vi "Create Database.vi"(8 "error in (no error)":errorcluster, 10 "Database Configuration":T1={"Interface"="CAN1", "CAN Cluster"={"Baud Rate"=125000, "Comment"="", "Name"="CAN_Cluster"}, "CAN Frame"={"Frame name"="frame1", "Identifier"=1, "Payload Length"=8, "Timing Type"=1, "Transmit Time"=0.0, "Extended Identifier?"=FALSE, "Comment"=""}, "Signal Cluster"={"Signal name"="signal", "Scaling Factor"=1.0, "Scaling Offset"=0.0, "Maximum Value"=256.0, "Minimum Value"=0.0, "Default Value"=0.0, "Unit"="V", "Start Bit"=0, "Number of Bits"=8, "Data Type"=1, "Byte Order"=0, "Comment"=""}, "Session Type (All Single Point)"=enum."Signal Input"} {"Signal Cluster"."Byte Order" items=["Little Endian", "Big Endian"]; "Signal Cluster"."Data Type" items=["Signed", "Unsigned", "IEEE Float"]; "CAN Frame"."Timing Type" items=["Cyclic Data", "Event Data", "Cyclic Remote", "Event Remote"]}, 11 "PXI 8513 in":refnum<class "PXI 8513.lvclass">) -> (0 "error out":errorcluster, 3 "PXI 8513 out":refnum<class "PXI 8513.lvclass">)   [LabVIEW 2016, in "CAN.lvlib" / "PXI 8513.lvclass"]
uses:
  PXI 8513.lvclass
  CAN Database Configuration.ctl
  C:/Program Files (x86)/National Instruments/LabVIEW 2016/examples/nixnet/examples.llb/NI-XNET Example Control - CAN Cluster.ctl
  C:/Program Files (x86)/National Instruments/LabVIEW 2016/examples/nixnet/examples.llb/NI-XNET Example Control - CAN Frame.ctl
  C:/Program Files (x86)/National Instruments/LabVIEW 2016/examples/nixnet/examples.llb/NI-XNET Example Control - Signal.ctl
  PXI 8513.lvclass/PXI 8513.ctl
  <vilib>/xnet/xnet.llb/XNET Create Session (Signal Input Single-point).vi
  <vilib>/xnet/xnet.llb/XNET Create Session (Signal Output Single-point).vi
  <vilib>/xnet/xnet.llb/XNET Create Session (Frame Input Single-point).vi
  <vilib>/xnet/xnet.llb/XNET Create Session (Frame Output Single-point).vi
  CAN.lvlib
panel:
  in  "Output Data":dbl=6.0 format="%.2f"
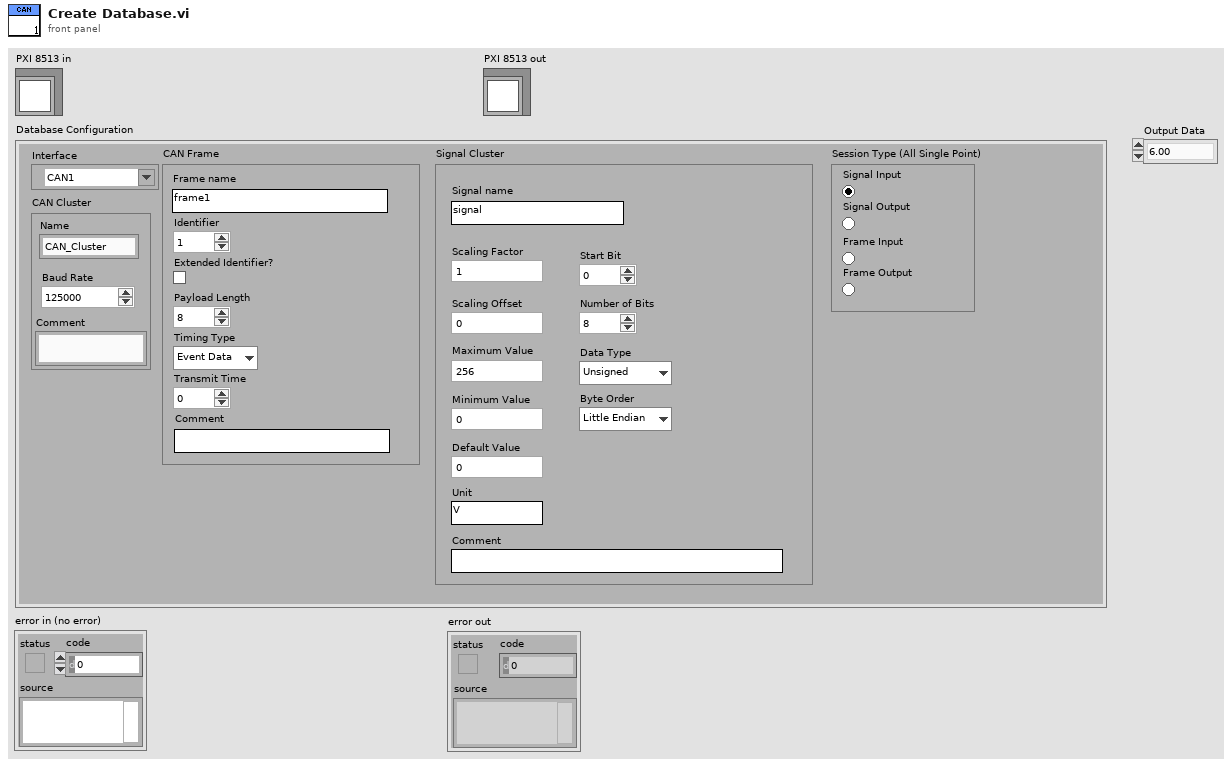
[diagram p1: front panel]
types:
  T1 = typedef "CAN.lvlib/CAN Database Configuration.ctl" = cluster{"Interface":refnum<k21>, "CAN Cluster":T2, "CAN Frame":T3, "Signal Cluster":T4, "Session Type (All Single Point)":enum32{"Signal Input", "Signal Output", "Frame Input", "Frame Output"}}
  T2 = typedef "NI-XNET Example Control - CAN Cluster.ctl" = cluster{"Baud Rate":u32, "Comment":string, "Name":string}
  T3 = typedef "NI-XNET Example Control - CAN Frame.ctl" = cluster{"Frame name":string, "Identifier":u32, "Payload Length":u32, "Timing Type":u32, "Transmit Time":dbl, "Extended Identifier?":bool, "Comment":string}
  T4 = typedef "NI-XNET Example Control - Signal.ctl" = cluster{"Signal name":string, "Scaling Factor":dbl, "Scaling Offset":dbl, "Maximum Value":dbl, "Minimum Value":dbl, "Default Value":dbl, "Unit":string, "Start Bit":u32, "Number of Bits":u32, "Data Type":u32, "Byte Order":u32, "Comment":string}
  T5 = enum32{"Signal Input", "Signal Output", "Frame Input", "Frame Output"}
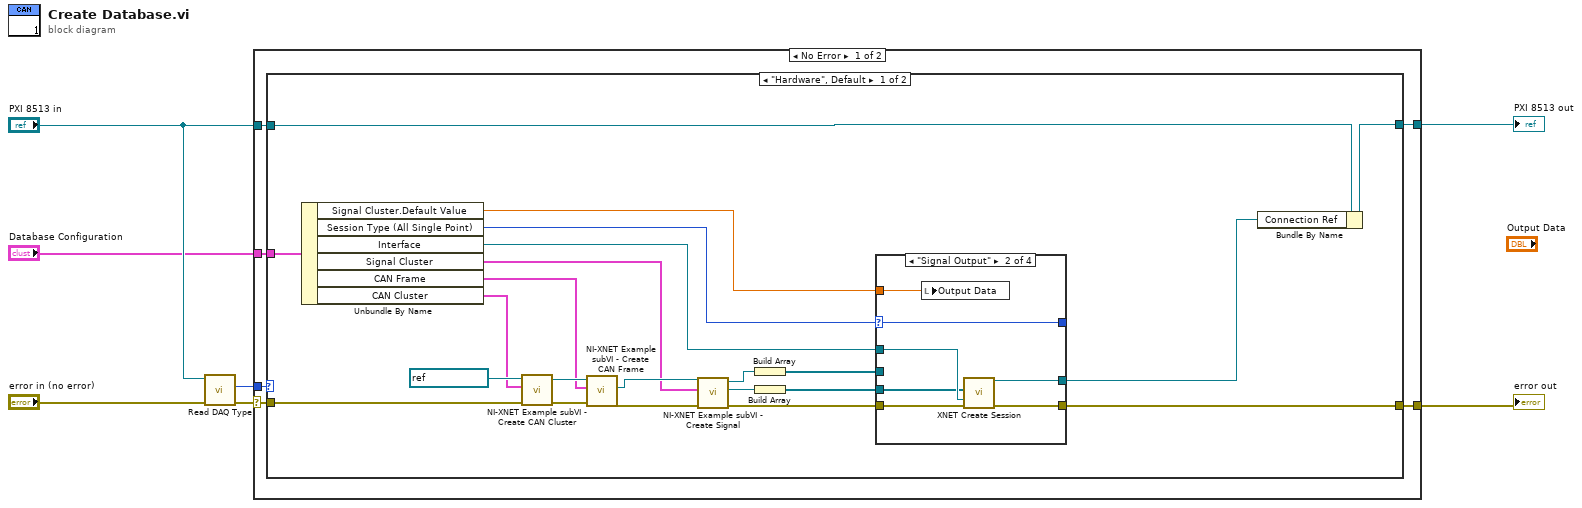
[diagram p0: block diagram]
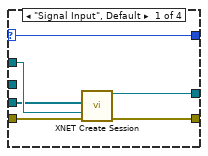
[diagram p2: hidden frame]
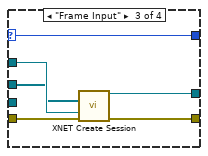
[diagram p3: hidden frame]
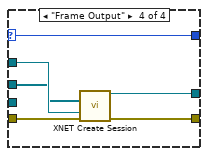
[diagram p4: hidden frame]
diagram:
  n1 = call-dynamic "Read DAQ Type.vi"("error in (no error)"="error in (no error)", "PXI 8513 in"="PXI 8513 in") -> ("error out"=w6:errorcluster, "DAQ Type"=w5:enum16{"Hardware", "Simulation"})  [unwired: 7 in, 1 out]
  n2 = case shown="No Error" w6 {
    selector: w6 -> [w10 w63]
    tunnel: w5 -> [w13 _]
    tunnel: "PXI 8513 in" -> [w12 w64]
    tunnel: "Database Configuration" -> [w11 _]
    tunnel: [w9 w63] -> w2
    tunnel: [w8 w64] -> w1
    frame No Error {
      n3 = case shown="\"Hardware\", Default" w13 {
        tunnel: w12 -> [w16 w62]
        tunnel: w11 -> [w29 _]
        tunnel: w10 -> [w30 w61]
        tunnel: [w17 w61] -> w9
        tunnel: [w15 w62] -> w8
        frame "Hardware", Default {
          n4 = Unbundle By Name(w29) -> ("Signal Cluster.Default Value"=w18:dbl, "Session Type (All Single Point)"=w24:T5, "Interface"=w23:refnum<k21>, "Signal Cluster"=w26:T4, "CAN Frame"=w27:T3, "CAN Cluster"=w28:T2)
          n5 = call "NI-XNET Example subVI - Create CAN Cluster.vi"("error in"=w30, "CAN Cluster"=w28, "database in"=refnum<k21> ":memory:" ("database in (:memory:)")) -> ("error out"=w34:errorcluster, "cluster out"=w33:refnum<k21>)  [unwired: 7 out]
          n6 = call "NI-XNET Example subVI - Create CAN Frame.vi"("error in"=w34, "CAN Frame"=w27, "cluster in"=w33) -> ("error out"=w35:errorcluster, "frame out"=w32:refnum<k21>)  [unwired: 3 in, 4 out]
          n7 = call "NI-XNET Example subVI - Create Signal.vi"("error in"=w35, "Signal Cluster"=w26, "frame in"=w32) -> ("error out"=w25:errorcluster, "signal out"=w20:refnum<k21>, "frame out"=w22:refnum<k21>)  [unwired: 6 out]
          n8 = Build Array(w22) -> (w21:refnum<k21>[])
          n9 = Build Array(w20) -> (w19:refnum<k21>[])
          n10 = case shown="\"Signal Output\"" w24 {
            selector: w24 -> [w38 w45 w52 w57]
            tunnel: w23 -> [w41 w48 w54 w58]
            tunnel: [w40 w47 w53 w59] -> w14
            tunnel: [w39 w46 w51 w60] -> w17
            tunnel: [w38 w45 w52 w57] -> _
            tunnel: w21 -> [_ _ w50 w56]
            tunnel: w25 -> [w37 w44 w49 w55]
            tunnel: w18 -> [_ w43 _ _]
            tunnel: w19 -> [w36 w42 _ _]
            frame "Signal Input", Default {
              n11 = call-poly <vilib>:"XNET Create Session.vi"("signal list"=w36, "interface"=w41, "error in (no error)"=w37) -> ("session out"=w40:refnum<k21>, "error out"=w39:errorcluster)  [unwired: 11 out]
            }
            frame "Signal Output" {
              n12 = local write "Output Data"(w43) -> ()
              n13 = call-poly <vilib>:"XNET Create Session.vi"("signal list"=w42, "interface"=w48, "error in (no error)"=w44) -> ("session out"=w47:refnum<k21>, "error out"=w46:errorcluster)  [unwired: 11 out]
            }
            frame "Frame Input" {
              n14 = call-poly <vilib>:"XNET Create Session.vi"("frame list"=w50, "interface"=w54, "error in (no error)"=w49) -> ("session out"=w53:refnum<k21>, "error out"=w51:errorcluster)  [unwired: 11 out]
            }
            frame "Frame Output" {
              n15 = call-poly <vilib>:"XNET Create Session.vi"("frame list"=w56, "interface"=w58, "error in (no error)"=w55) -> ("session out"=w59:refnum<k21>, "error out"=w60:errorcluster)  [unwired: 11 out]
            }
          }
          n16 = Bundle By Name(cluster=w16, "Connection Ref"=w14) -> (w15:refnum<class "PXI 8513.lvclass">)
        }
        frame "Simulation" {
        }
      }
    }
    frame Error {
    }
  }
  "error out" <- w2
  "PXI 8513 out" <- w1
